vi "Send command Set Pin.vi"(0 "Serial Device in":refnum<class "Serial Device.lvclass">, 1 "Puerto":string(combo), 2 "Pin":string(combo), 3 "Valor":string(combo), 5 "error in (no error)":errorcluster, 6 "Marca":string) -> (14 "Serial Device out":refnum<class "Serial Device.lvclass">, 16 "Command":string, 17 "Expected response":string, 19 "error out":errorcluster)   [LabVIEW 2020, in "Serial Device.lvclass"]
uses:
  Serial Device.lvclass
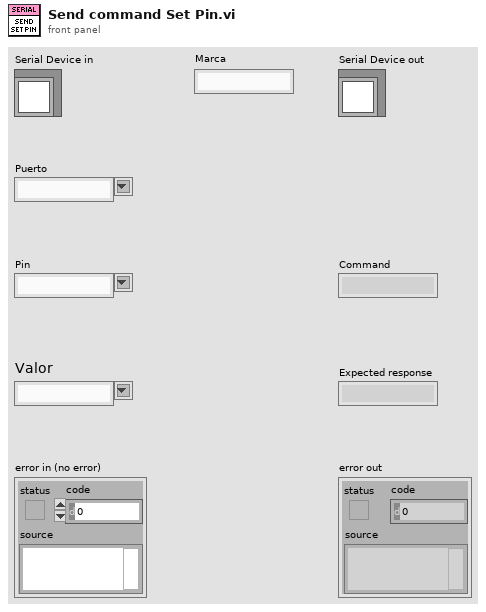
[diagram p1: front panel]
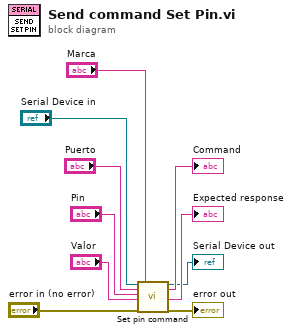
[diagram p0: block diagram]
diagram:
  n1 = call-dynamic "Set pin command.vi"("Serial Device in"="Serial Device in", "Puerto"="Puerto", "Pin"="Pin", "Valor"="Valor", "error in (no error)"="error in (no error)", "Marca"="Marca") -> ("Serial Device out"=→"Serial Device out":refnum<class "Serial Device.lvclass">, "Command"=→"Command":string, "Expected response"=→"Expected response":string, "error out"=→"error out":errorcluster)  [unwired: 10 in]
